vi "CH_LM DFM Catalog.vi"(0 "Meter Index":i32, 5 "error in (no error)":errorcluster, 7 "Timeout / ms (3000)":i32=3000, 9 "Lock Timeout / ms (1000)":i32=1000) -> (11 "Lock timed out":bool, 14 "Meter Index":i32, 15 "Bytes in use":i32, 16 "Bytes available":i32, 17 "Catalog":T1[](array[typedef]), 19 "error out":errorcluster)   [LabVIEW 2012, in "CH_LM.lvlib"]
doc: "This query will get trend data file mass storage information and a list of trend data files stored in the current working directory. The file size in bytes is an estimated value in the case of active open files.\n\n<B>Note:</B> SCPI specifies using the term \"catalog\" in lieu of the term \"directory\" as the header to request a list of files contained in a directory. In that context, catalog and directory are synonymous.\n\n<B>Attention:</B> This VI contains a work arround because the file list is returned in several respoce records and not one single."
uses:
  CH_LM.lvlib
  CH_LM File Information.ctl
panel:
  in  "NofStrings (-1:all)":i32=-1
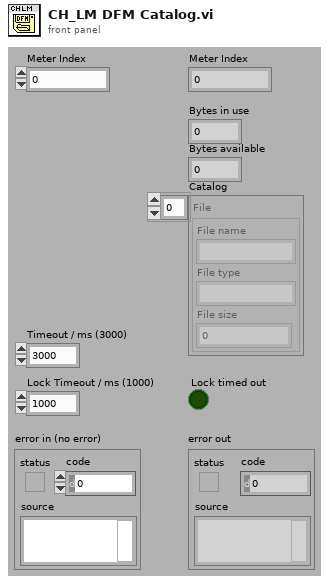
[diagram p1: front panel]
types:
  T1 = typedef "CH_LM.lvlib/CH_LM File Information.ctl" = cluster{"File name":string, "File type":string, "File size":i32}
  T2 = cluster{"trimmed string":string, "trimmed string":string, i32}
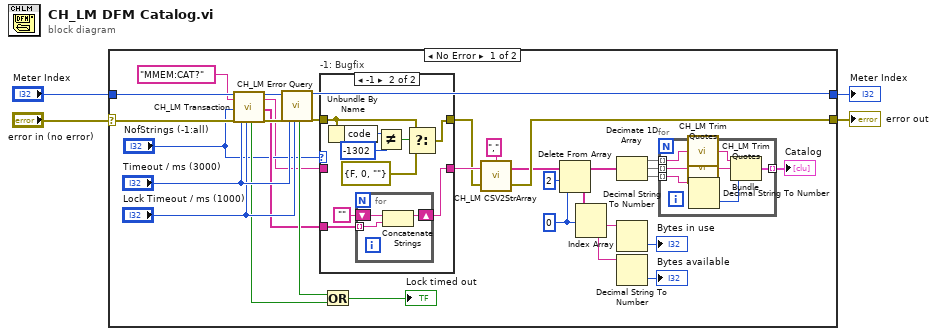
[diagram p0: block diagram]
diagram:
  n1 = case shown="No Error" "error in (no error)" {
    selector: "error in (no error)" -> [w36 w59]
    tunnel: [w25 w59] -> w4
    tunnel: "Meter Index" -> [w35 w58]
    tunnel: [w31 w58] -> w1
    frame No Error {
      w22 = 0 ("index")
      n2 = call "CH_LM Transaction.vi"("Meter Index"=w35, "Command String"="MMEM:CAT?", "NofStrings (-1:all)"="NofStrings (-1:all)", "error in (no error)"=w36, "Timeout / ms (3000)"="Timeout / ms (3000)", "Lock Timeout / ms (1000)"="Lock Timeout / ms (1000)") -> ("Lock timed out"=w27:bool, "Meter Index"=w32:i32, "Response"=w8:string, "Response Array"=w11:string[], "error out"=w33:errorcluster)  [unwired: 9 out]
      n3 = call "CH_LM Error Query.vi"("Meter Index"=w32, "error in (no error)"=w33, "Timeout / ms (3000)"="Timeout / ms (3000)", "Lock Timeout / ms (1000)"="Lock Timeout / ms (1000)") -> ("Lock timed out"=w28:bool, "Meter Index"=w31:i32, "error out"=w6:errorcluster)  [unwired: 13 out]
      n4 = case "-1: Bugfix" shown="-1" "NofStrings (-1:all)" {
        tunnel: w11 -> [_ w47]
        tunnel: [w38 w45] -> w9
        tunnel: w8 -> [w38 _]
        tunnel: w6 -> [w37 w41]
        tunnel: [w37 w40] -> w5
        frame 0, Default {
        }
        frame -1 {
          n5 = Unbundle By Name(w41) -> ("code"=w44:i32)
          n6 = for {
            tunnel: w47 -> [w49] mode=indexing
            shift-right: [w48] -> w45
            shift-left: "" -> [w50]
            n7 = Concatenate Strings(w50, w49) -> (w48:string)
          }
          n8 = Not Equal?(x=w44, y=-1302) -> (x != y?=w42:bool)
          n9 = Select(t=w41, s=w42, f=errorcluster {"status"=FALSE, "code"=0, "source"=""}) -> (s? t:f=w40:errorcluster)
        }
      }
      n10 = Or(x=w28, y=w27) -> (x .or. y?=→"Lock timed out":bool)
      n11 = call "CH_LM CSV2StrArray.vi"("error in (no error)"=w5, "CSL"=w9, "Separator (,)"=",") -> ("error out"=w25:errorcluster, "Strings"=w18:string[])
      n12 = Delete From Array(array=w18, length=2, index=w22) -> (deleted portion=w23:string[], array with subset deleted=w17:string[])
      n13 = Index Array(array=w23, index #1=w22) -> (element #1=w21:string, element #2=w7:string)  [unwired: 1 in]
      n14 = Decimate 1D Array(w17) -> (w16:string[], w15:string[], w14:string[])
      n15 = Decimal String To Number(string=w21) -> (number=→"Bytes in use":i32)  [unwired: 3 out]
      n16 = Decimal String To Number(string=w7) -> (number=→"Bytes available":i32)  [unwired: 3 out]
      n17 = for {
        tunnel: w16 -> [w54] mode=indexing
        tunnel: w15 -> [w51] mode=indexing
        tunnel: w14 -> [w57] mode=indexing
        tunnel: [w55] -> w13 mode=indexing
        n18 = call "CH_LM Trim Quotes.vi"("string"=w54) -> ("trimmed string"=w53:string)  [unwired: 1 in]
        n19 = call "CH_LM Trim Quotes.vi"("string"=w51) -> ("trimmed string"=w52:string)  [unwired: 1 in]
        n20 = Decimal String To Number(string=w57) -> (number=w56:i32)  [unwired: 3 out]
        n21 = Bundle("trimmed string"=w53, "trimmed string"=w52, w56) -> (w55:T2)  [unwired: 1 out]
      }
      "Catalog" <- w13
    }
    frame Error {
    }
  }
  "error out" <- w4
  "Meter Index" <- w1
